vi "GET ARM STATUS.vi"(8 "error in (no error)":errorcluster, 9 "SOLENOID refnum name":string="My Solenoid RefNum", 10 "MOTOR refnum name":string="My Motor RefNum", 11 "SIDE":enum16{"LEFT", "RIGHT"}(ring)) -> (0 "error out":errorcluster, 1 "Sensor Position":dbl, 2 "RETRACT Limit?":bool, 3 "EXTEND Limit?":bool)   [LabVIEW 2023]
uses:
  <vilib>/Rock Robotics/WPI/Solenoid/Deprecated/WPI_SolenoidGetBool.vi
  <vilib>/Rock Robotics/Network Tables/NT Write Boolean.vi
  Global odometry.vi
  <vilib>/Rock Robotics/Network Tables/NT Write Number.vi
panel:
  in  "STACK BASE":string
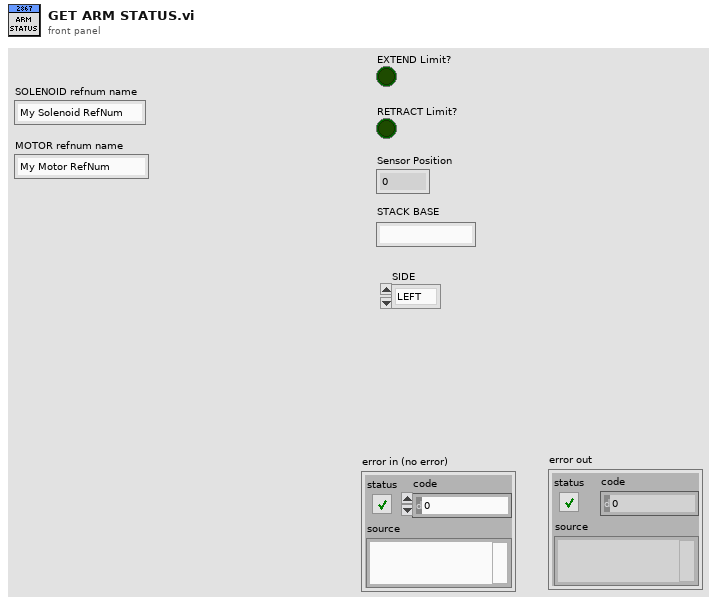
[diagram p1: front panel]
types:
  T1 = typedef "WPI_SolenoidDevRef.ctl" = cluster{"DevStatus":errorcluster, "Pneumatics Control Module":u8, "Forward Solenoid Channel":T2, "Reverse Solenoid Channel":T2}
  T2 = typedef "WPI_SolenoidChannel.ctl" = enum8{"Solenoid 0", "Solenoid 1", "Solenoid 2", "Solenoid 3", "Solenoid 4", "Solenoid 5", "Solenoid 6", "Solenoid 7", "Solenoid 8", "Solenoid 9", "Solenoid 10", "Solenoid 11", "Solenoid 12", "Solenoid 13", "Solenoid 14", "Solenoid 15", "Invalid"}
  T3 = typedef "WPI_MotorControlDeviceRef.ctl" = cluster{"DeviceStatus":errorcluster, "Type":T4, "PWM":cluster{"PWM Channel":T5, "DeadBand":T6}, "CAN":cluster{"Device Number":u8, "SetOutput VI Ref":variant, "GetOutput VI Ref":variant, "Enable VI Ref":variant, "Disable VI Ref":variant, "Data":variant}, "Invert":bool, "DIO PWM":cluster{"PWM \"Enable\" Channel":T5, "DIOChannel":T7, "PWM Rate":dbl}}
  T4 = typedef "WPI_MotorControlType.ctl" = enum16{"PWM", "CAN", "DIO PWM"}
  T5 = typedef "FPGA_DIOPWMChannel.ctl" = enum8{"PWM 0", "PWM 1", "PWM 2", "PWM 3", "PWM 4", "PWM 5", "PWM 6", "PWM 7", "PWM 8", "PWM 9", "PWM MXP 0", "PWM MXP 1", "PWM MXP 2", "PWM MXP 3", "PWM MXP 4", "PWM MXP 5", "PWM MXP 6", "PWM MXP 7", "PWM MXP 8", "PWM MXP 9", "Invalid"}
  T6 = typedef "WPI_PWMDeadband.ctl" = cluster{"Name":string, "maxPositivePwm":i32, "minPositivePwm":i32, "centerPwm":i32, "maxNegativePwm":i32, "minNegativePwm":i32, "angularRange":u16}
  T7 = typedef "FPGA_DIOChannel.ctl" = enum8{"DIO 0", "DIO 1", "DIO 2", "DIO 3", "DIO 4", "DIO 5", "DIO 6", "DIO 7", "DIO 8", "DIO 9", "DIO MXP 0", "DIO MXP 1", "DIO MXP 2", "DIO MXP 3", "DIO MXP 4", "DIO MXP 5", "DIO MXP 6", "DIO MXP 7", "DIO MXP 8", "DIO MXP 9", "DIO MXP 10", "DIO MXP 11", "DIO MXP 12", "DIO MXP 13", "DIO MXP 14", "DIO MXP 15", "SPI Port CS1", "SPI Port CS2", "SPI Port CS3", "SPI Port MISO", "SPI Port MOSI", "Invalid"}
  T8 = cluster{"LEFT ARM":cluster{"VBus%":dbl, "LOCK?":bool, "LOCKED":bool}, "RIGHT ARM":cluster{"VBus%":dbl, "LOCK?":bool, "LOCKED":bool}}
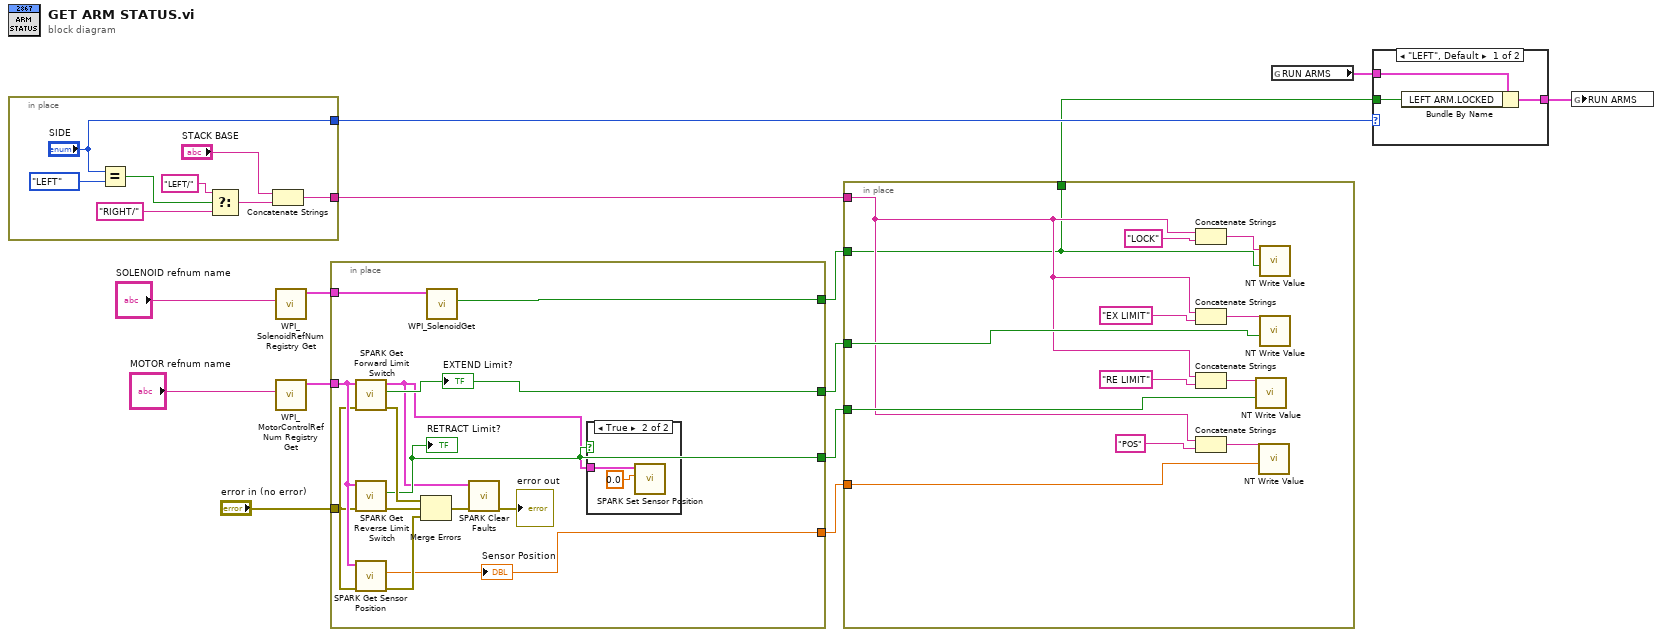
[diagram p0: block diagram]
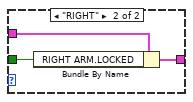
[diagram p2: hidden frame]
diagram:
  n1 = in-place {
    in-place-border: [w16] -> w9
    in-place-border: ["SIDE"] -> w8
    n2 = Equal?(x="SIDE", y=enum16{"LEFT", "RIGHT"}."LEFT") -> (x = y?=w21:bool)
    n3 = Select(t="LEFT/", s=w21, f="RIGHT/") -> (s? t:f=w18:string)
    n4 = Concatenate Strings("STACK BASE", w18) -> (w16:string)
  }
  n5 = call <vilib>:"WPI_SolenoidRefNum Registry Get.vi"("refnum name"="SOLENOID refnum name") -> ("SolenoidDevRef"=w2:T1)  [unwired: 9 in, 1 out]
  n6 = call <vilib>:"WPI_MotorControlRefNum Registry Get.vi"("refnum name"="MOTOR refnum name") -> ("MotorControlDevRef"=w4:T3)  [unwired: 9 in, 1 out]
  n7 = in-place {
    in-place-border: w4 -> [w34]
    in-place-border: "error in (no error)" -> [w33]
    in-place-border: w2 -> [w31]
    in-place-border: [w27] -> w13
    in-place-border: [w24] -> w12
    in-place-border: [w26] -> w11
    in-place-border: [w25] -> w10
    n8 = call <vilib>:"SPARK Get Forward Limit Switch.vi"("error in (no error)"=w33, "MotorControlDevRef in"=w34) -> ("error out"=w30:errorcluster, "Hard Limit Fwd"=w26:bool, "MotorControlDevRef out"=w23:T3)  [unwired: 6 in, 1 out]
    "EXTEND Limit?" <- w26
    n9 = call <vilib>:"SPARK Get Reverse Limit Switch.vi"("error in (no error)"=w33, "MotorControlDevRef in"=w34) -> ("error out"=w29:errorcluster, "Hard Limit Rev"=w24:bool)  [unwired: 6 in, 2 out]
    "RETRACT Limit?" <- w24
    n10 = call <vilib>:"SPARK Get Sensor Position.vi"("error in (no error)"=w33, "MotorControlDevRef in"=w34) -> ("error out"=w28:errorcluster, "Sensor Position"=w27:dbl)  [unwired: 6 in, 2 out]
    "Sensor Position" <- w27
    n11 = Merge Errors(w30, w29, w28) -> (w35:errorcluster)
    n12 = call-poly <vilib>:"WPI_SolenoidGet.vi"("SolenoidDevRef"=w31) -> ("Value"=w25:bool)  [unwired: 8 in, 2 out]
    n13 = call <vilib>:"SPARK Clear Faults.vi"("error in"=w35, "MotorControlDeviceRef"=w23) -> ("error out"=→"error out":errorcluster)  [unwired: 8 in, 1 out]
    n14 = case shown="True" w24 {
      tunnel: w23 -> [_ w36]
      frame False {
      }
      frame True {
        n15 = call <vilib>:"SPARK Set Sensor Position.vi"("Position"=0.0, "MotorControlDeviceRef"=w36) -> ()  [unwired: 8 in, 2 out]
      }
    }
  }
  n16 = in-place {
    in-place-border: w13 -> [w50]
    in-place-border: w12 -> [w49]
    in-place-border: w11 -> [w48]
    in-place-border: w10 -> [w38]
    in-place-border: w9 -> [w39]
    in-place-border: [w38] -> w5
    n17 = Concatenate Strings(w39, "LOCK" ("ARM LOCK")) -> (w47:string)
    n18 = Concatenate Strings(w39, "EX LIMIT" ("ARM EXTEND")) -> (w46:string)
    n19 = Concatenate Strings(w39, "RE LIMIT" ("ARM RETRACT")) -> (w45:string)
    n20 = Concatenate Strings(w39, "POS" ("ARM LIMIT EXTEND")) -> (w44:string)
    n21 = call-poly <vilib>:"NT Write Value.vi"("value"=w49, "name"=w45) -> ()  [unwired: 9 in, 1 out]
    n22 = call-poly <vilib>:"NT Write Value.vi"("value"=w50, "name"=w44) -> ()  [unwired: 9 in, 1 out]
    n23 = call-poly <vilib>:"NT Write Value.vi"("value"=w38, "name"=w47) -> ()  [unwired: 9 in, 1 out]
    n24 = call-poly <vilib>:"NT Write Value.vi"("value"=w48, "name"=w46) -> ()  [unwired: 9 in, 1 out]
  }
  n25 = global read "Global odometry.vi" "RUN ARMS"() -> (w7:T8)
  n26 = case shown="\"LEFT\", Default" w8 {
    tunnel: w7 -> [w52 w56]
    tunnel: [w53 w55] -> w6
    tunnel: w5 -> [w51 w54]
    frame "LEFT", Default {
      n27 = Bundle By Name(cluster=w52, "LEFT ARM.LOCKED"=w51) -> (w53:T8)
    }
    frame "RIGHT" {
      n28 = Bundle By Name(cluster=w56, "RIGHT ARM.LOCKED"=w54) -> (w55:T8)
    }
  }
  n29 = global write "Global odometry.vi" "RUN ARMS"(w6) -> ()
